vi "ConvertArray.vi"(11 "Data In":u8[](array[numeric])) -> (3 "Data Out":u16[](array[numeric]))   [LabVIEW 2009]
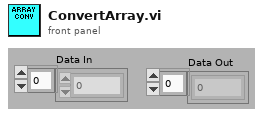
[diagram p1: front panel]
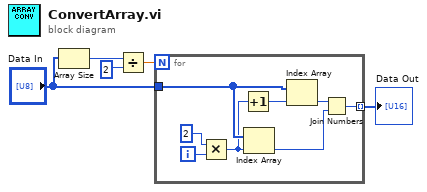
[diagram p0: block diagram]
diagram:
  n1 = Array Size(array="Data In") -> (size(s)=w5:i32)
  n2 = Divide(x=w5, y=2) -> (x/y=w3:dbl)
  n3 = for {
    N: w3 -> [_]
    tunnel: "Data In" -> [w13]
    tunnel: [w6] -> w1 mode=indexing
    i -> [w12]
    n4 = Multiply(x=2, y=w12) -> (x*y=w9:i32)
    n5 = Increment(x=w9) -> (x+1=w10:i32)
    n6 = Index Array(array=w13, index=w9) -> (element=w7:u8)
    n7 = Index Array(array=w13, index=w10) -> (element=w8:u8)
    n8 = Join Numbers(hi=w8, lo=w7) -> ((hi.lo)=w6:u16)
  }
  "Data Out" <- w1
